vi "StartClone.vi"(7 "ShowPanel? (f)":bool, 8 "error in (no error)":errorcluster, 10 "ModuleName":string="unnamed", 11 "VI Refnum":refnum<vi>) -> (0 "error out":errorcluster, 1 "clBroadcastEvents":T1, 3 "ModuleAdmin":refnum<class "ModuleAdmin.lvclass">)   [LabVIEW 2018, in "MyPluggableModule.lvlib"]
uses:
  MyPluggableModule.lvlib
  PluginsShared/clBroadcastEvents.ctl
  PluginsShared/clEventType.ctl
  <userlib>/NIST/ModuleAdminLib/ModuleAdmin/ModuleAdmin.lvclass
  C:/Program Files (x86)/National Instruments/LabVIEW 2018/user.lib/NIST/ModuleAdminLib/ModuleAdminBase/ModuleAdminBase.lvclass
  <userlib>/NIST/ModuleAdminLib/ModuleAdmin/ModuleAdmin.lvclass/ModuleAdmin.ctl
  <userlib>/NIST/ModuleAdminLib/ModuleAdmin/Accessors/Write CloneRegRef.vi
  <userlib>/NIST/ModuleAdminLib/ModuleAdmin/Accessors/Write ShowPanel_.vi
  <vilib>/Utility/error.llb/Error Cluster From Error Code.vi
  <vilib>/ErrorRing/Error Ring.xnode
  PluginsShared/PluginsShared.lvlib
  <userlib>/NIST/ModuleAdminLib/ModuleAdminBase/ModuleAdminBase.lvclass
  <userlib>/NIST/ModuleAdminLib/CloneRegistration/CloneRegistration.lvclass
panel:
  # "If you want to add other Broadcast Events, open this typedef, copy an existing event and rename it to your event name.\n\nNext create an \"arg\" typedef for the  data and put it into PublicAPI/Arguments/Broadcasts\n\nAfter that, you will need to create a new roadcast vi in Protected/Broadcast.  Look at DidInit.vi or the reportError.vi as examples."
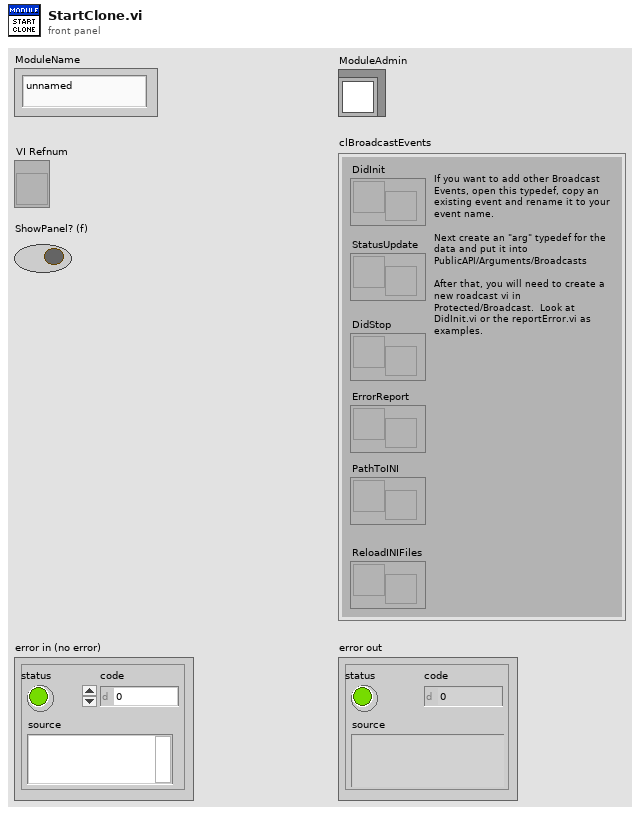
[diagram p1: front panel]
types:
  T1 = typedef "PluginsShared.lvlib/clBroadcastEvents.ctl" = cluster{"DidInit":refnum<user-event>, "StatusUpdate":refnum<user-event>, "ErrorReport":refnum<user-event>, "DidStop":refnum<user-event>, "PathToINI":refnum<user-event>, "ReloadINIFiles":refnum<user-event>}
  T2 = enum32{"Bad", "Idle", "Run top level", "Running"}
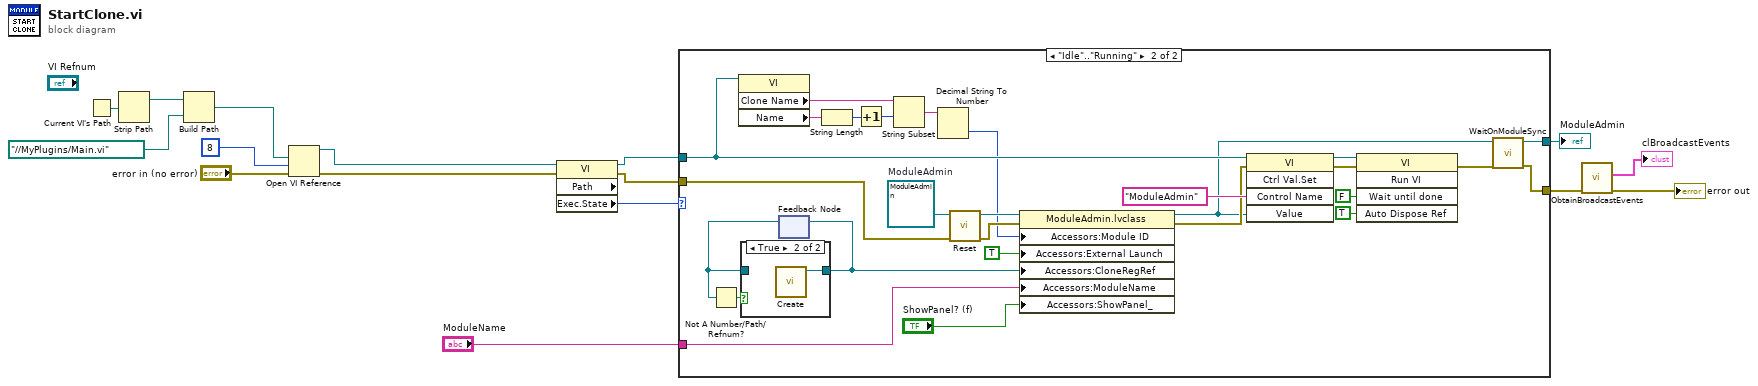
[diagram p0: block diagram]
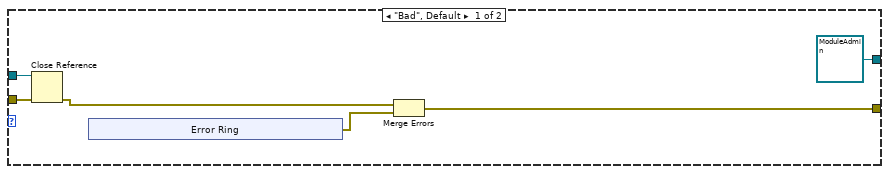
[diagram p2: hidden frame]
diagram:
  n1 = Current VI's Path() -> (path=w8:path)
  n2 = Strip Path(path=w8) -> (stripped path=w9:path)  [unwired: 1 out]
  n3 = Build Path(base path=w9, name or relative path=path "../../MyPlugins/Main.vi" ("vi path")) -> (appended path=w6:path)
  n4 = Open VI Reference(vi path=w6, options=8, error in (no error)="error in (no error)") -> (vi reference=w3:refnum<vi>, error out=w5:errorcluster)  [unwired: 3 in]
  n5 = property class="VI" props=["Path", "Exec.State"](reference=w3, error in=w5) -> (reference out=w2:refnum<vi>, error out=w4:errorcluster, "Exec.State"=w16:T2)  [unwired: 1 out]
  n6 = case shown="\"Idle\"..\"Running\"" w16 {
    tunnel: w4 -> [w22 w27]
    tunnel: w2 -> [w21 w44]
    tunnel: [w18 w34] -> w14
    tunnel: "ModuleName" -> [_ w33]
    tunnel: [refnum<class "ModuleAdmin.lvclass"> refnum ("ModuleAdmin") w32] -> w12
    frame "Bad", Default {
      n7 = Close Reference(reference=w21, error in (no error)=w22) -> (error out=w20:errorcluster)
      n8 = xnode "Error Ring"() -> ("error out"=w19:errorcluster)
      n9 = Merge Errors(w20, w19) -> (w18:errorcluster)
    }
    frame "Idle".."Running" {
      w48 = refnum<class "ModuleAdmin.lvclass"> refnum  # ModuleAdmin
      n10 = property class="VI"(reference=w44) -> ("Clone Name"=w50:string, "Name"=w53:string)  [unwired: 1 in, 2 out]
      n11 = feedback #1() -> (w29:refnum<data-value>)  [unwired: 1 in]
      n12 = Not A Number/Path/Refnum?(number/path/refnum=w29) -> (NaN/Path/Refnum?=w30:bool)
      n13 = case shown="True" w30 {
        tunnel: [w54 w55] -> w28
        tunnel: w29 -> [w54 _]
        frame False {
        }
        frame True {
          n14 = call <userlib>:"Create.vi"() -> ("CloneRegRef"=w55:refnum<data-value>)  [unwired: 10 in, 1 out]
        }
      }
      n15 = feedback-in #1(w28) -> ()
      n16 = String Length(string=w53) -> (length=w52:i32)
      n17 = Increment(x=w52) -> (x+1=w51:i32)
      n18 = String Subset(string=w50, offset (0)=w51) -> (substring=w49:string)  [unwired: 1 in]
      n19 = Decimal String To Number(string=w49) -> (number=w36:i32)  [unwired: 2 in, 1 out]
      n20 = call <userlib>:"Reset.vi"("error in (no error)"=w27, "Mod Admin in"=w48) -> ("error out"=w47:errorcluster, "Mod Admin out"=w46:refnum<class "ModuleAdmin.lvclass">)  [unwired: 8 in]
      n21 = property class="ModuleAdmin.lvclass"(reference=w46, error in=w47, "Accessors:Module ID"=w36, "Accessors:External Launch"=TRUE ("External Launch"), "Accessors:CloneRegRef"=w28, "Accessors:ModuleName"=w33, "Accessors:ShowPanel_"="ShowPanel? (f)") -> (reference out=w35:refnum<class "ModuleAdmin.lvclass">, error out=w37:errorcluster)
      n22 = invoke class="VI" method="Ctrl Val.Set"(reference=w44, error in=w37, "Control Name"="ModuleAdmin", "Value"=w35) -> (reference out=w42:refnum<vi>, error out=w41:errorcluster)  [unwired: 1 in, 3 out]
      n23 = invoke class="VI" method="Run VI"(reference=w42, error in=w41, "Wait until done"=FALSE ("Wait Until Done"), "Auto Dispose Ref"=TRUE ("Auto Dispose Reference")) -> (error out=w38:errorcluster)  [unwired: 1 in, 4 out]
      n24 = call <userlib>:"WaitOnModuleSync.vi"("error in (no error)"=w38, "ModuleAdmin"=w35) -> ("error out"=w34:errorcluster, "ModuleAdmin"=w32:refnum<class "ModuleAdmin.lvclass">)  [unwired: 8 in]
    }
  }
  "ModuleAdmin" <- w12
  n25 = call "ObtainBroadcastEvents.vi"("error in (no error)"=w14) -> ("error out"=→"error out":errorcluster, "clBroadcastEvents"=→"clBroadcastEvents":T1)  [unwired: 9 in]
